vi "Curtin1_RenameFIles.vi"(8 "Files and folders?":bool=TRUE, 9 "Old Name":string, 10 "New Name":string, 11 "Path To Test Folder":path) -> ()   [LabVIEW 2022 SP3]
panel:
  out "error out":errorcluster
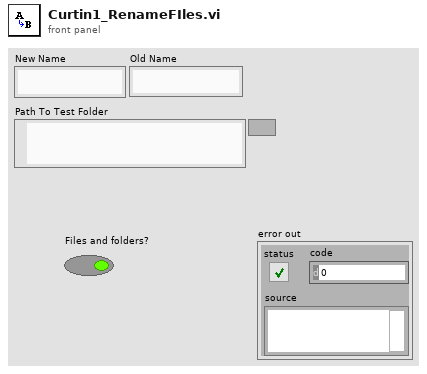
[diagram p1: front panel]
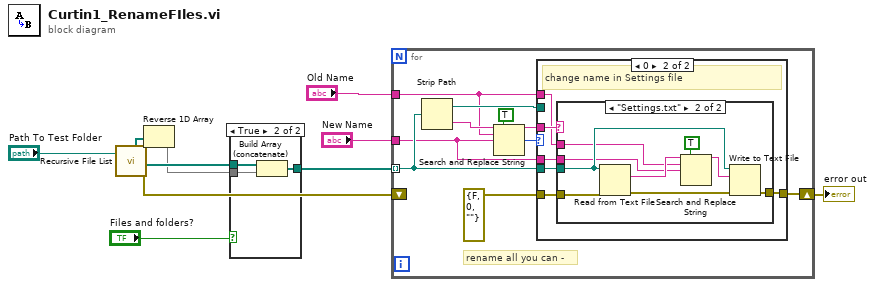
[diagram p0: block diagram]
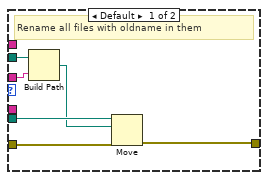
[diagram p3: hidden frame]
diagram:
  n1 = call <vilib>:"Recursive File List.vi"("Folder Path"="Path To Test Folder") -> ("error out"=w6:errorcluster, "All Files in Dir"=w3:path[], "All Folders"=w9:path[])  [unwired: 6 in, 2 out]
  n2 = Reverse 1D Array(array=w9) -> (reversed array=w2:path[])
  n3 = case shown="True" "Files and folders?" {
    tunnel: [w11 w14] -> w4
    tunnel: w3 -> [w11 w13]
    tunnel: w2 -> [_ w12]
    frame False {
    }
    frame True {
      n4 = Build Array (concatenate)(w13, w12) -> (w14:path[])
    }
  }
  n5 = for {
    tunnel: w4 -> [w21] mode=indexing
    tunnel: "Old Name" -> [w17]
    tunnel: "New Name" -> [w18]
    shift-right: [w16] -> w5
    shift-left: w6 -> [_]
    # "rename all you can -"
    n6 = Strip Path(path=w21) -> (stripped path=w19:path, name=w24:string)
    n7 = Search and Replace String(replace all?=TRUE ("replace all? (F)"), input string=w24, search string=w17, replace string=w18) -> (result string=w20:string, number of replacements=w22:i32)  [unwired: 4 in, 2 out]
    n8 = case shown="0" w22 {
      tunnel: w21 -> [w30 w35]
      tunnel: w20 -> [w29 w36]
      tunnel: w19 -> [w28 _]
      tunnel: w18 -> [_ w34]
      tunnel: w17 -> [_ w33]
      tunnel: [w26 w32] -> w16
      tunnel: errorcluster {"status"=FALSE, "code"=0, "source"=""} ("error out") -> [w25 w31]
      frame Default {
        # "Rename all files with oldname in them"
        n9 = Build Path(base path=w28, name or relative path=w29) -> (appended path=w27:path)
        n10 = Move(source path=w30, error in=w25, 10:w27) -> (error out=w26:errorcluster)  [unwired: 2 in, 2 out]
      }
      frame 0 {
        # "change name in Settings file"
        n11 = case shown="\"Settings.txt\"" w36 {
          tunnel: w35 -> [_ w46]
          tunnel: w34 -> [_ w41]
          tunnel: w33 -> [_ w40]
          tunnel: [w37 w39] -> w32
          tunnel: w31 -> [w37 w38]
          frame Default {
          }
          frame "Settings.txt" {
            n12 = Read from Text File(file (use dialog)=w46, error in=w38) -> (text=w45:string, error out=w43:errorcluster)  [unwired: 2 in, 2 out]
            n13 = Search and Replace String(replace all?=TRUE ("replace all? (F)"), input string=w45, search string=w40, replace string=w41) -> (result string=w44:string)  [unwired: 4 in, 3 out]
            n14 = Write to Text File(file (use dialog)=w46, text=w44, error in=w43) -> (error out=w39:errorcluster)  [unwired: 1 in, 2 out]
          }
        }
      }
    }
  }
  "error out" <- w5
